vi "Calc Init.vi"(8 "error in (no error)":errorcluster, 10 "Config":refnum<class "Channel Config.lvclass">, 11 "Div Calc in":refnum<class "Div Calc.lvclass">) -> (0 "error out":errorcluster, 3 "Div Calc out":refnum<class "Div Calc.lvclass">)   [LabVIEW 2020, in "VolatusCalcs.lvlib" / "Div Calc.lvclass"]
uses:
  Div Calc.lvclass
  Div Calc.lvclass/Div Calc.ctl
  VolatusConfig/VolatusConfigElement/VolatusConfigElement.lvclass
  lv-cdm/CDM-Config/Config Element/Config Element.lvclass
  VolatusConfig/Channel/Channel Config.lvclass
  C:/dev/lv20CE/relink/lv-volatus/VolatusConfig/VolatusConfigElement/VolatusConfigElement.lvclass
  C:/dev/lv20CE/relink/lv-volatus/VolatusConfig/Channel/Channel Config.lvclass
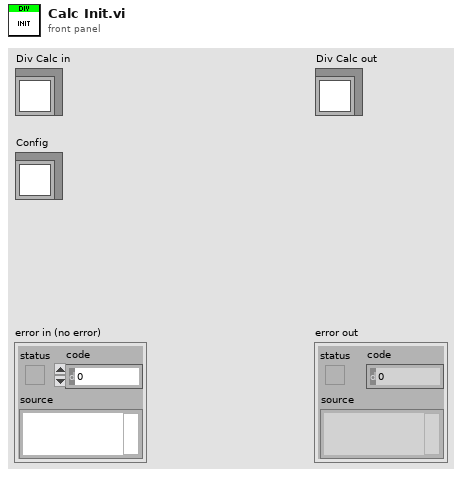
[diagram p1: front panel]
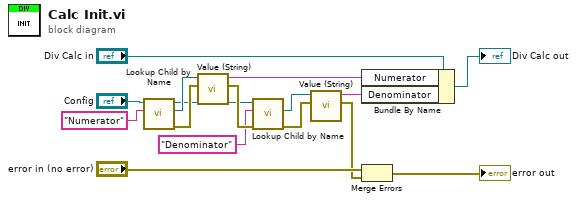
[diagram p0: block diagram]
diagram:
  n1 = call "Lookup Child by Name.vi"("Child Name"="Numerator", "VolatusConfigElement in"="Config") -> ("error out"=w9:errorcluster, "Child"=w10:refnum<class "Config Element.lvclass">, "VolatusConfigElement out"=w1:refnum<class "Channel Config.lvclass">)  [unwired: 6 in, 1 out]
  n2 = call "Value (String).vi"("error in (no error)"=w9, "Config Element in"=w10) -> ("error out"=w16:errorcluster, "String Value"=w4:string)  [unwired: 8 in]
  n3 = call "Lookup Child by Name.vi"("error in (no error)"=w16, "Child Name"="Denominator", "VolatusConfigElement in"=w1) -> ("error out"=w7:errorcluster, "Child"=w8:refnum<class "Config Element.lvclass">)  [unwired: 5 in, 2 out]
  n4 = call "Value (String).vi"("error in (no error)"=w7, "Config Element in"=w8) -> ("error out"=w2:errorcluster, "String Value"=w5:string)  [unwired: 8 in]
  n5 = Bundle By Name(cluster="Div Calc in", "Numerator"=w4, "Denominator"=w5) -> (→"Div Calc out":refnum<class "Div Calc.lvclass">)
  n6 = Merge Errors("error in (no error)", w2) -> (→"error out":errorcluster)
